vi "Public Pass.vi"(7 "Description":string, 8 "error in (no error)":errorcluster, 9 "Message":string, 11 "Test Case Test Double in":refnum<class "Test Case Test Double.lvclass">) -> (0 "error out":errorcluster, 3 "Test Case Test Double out":refnum<class "Test Case Test Double.lvclass">)   [LabVIEW 2020, in "Test Case Test Double.lvclass"]
uses:
  Test Case Test Double.lvclass
  source/Framework/Test Case/LUnit Test Case.lvclass
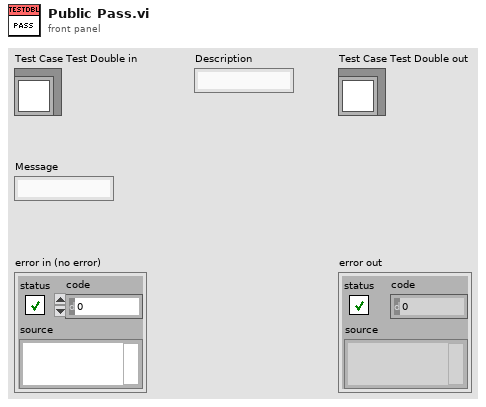
[diagram p1: front panel]
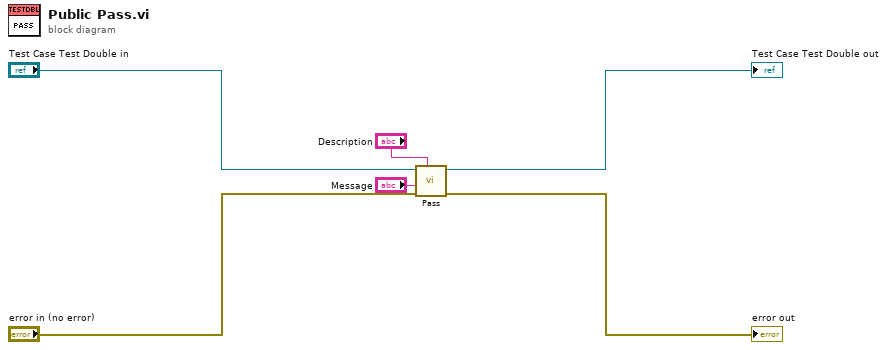
[diagram p0: block diagram]
diagram:
  n1 = call "Pass.vi"("Description"="Description", "error in (no error)"="error in (no error)", "Message"="Message", "LUnit Test Case In"="Test Case Test Double in") -> ("error out"=→"error out":errorcluster, "LUnit Test Case Out"=→"Test Case Test Double out":refnum<class "Test Case Test Double.lvclass">)  [unwired: 6 in]
